vi "Get ESC Ready.vi"(3 "Error in":errorcluster) -> (0 "Error out":errorcluster, 2 "Current PWM%":dbl)   [LabVIEW 2021]
uses:
  Anemometry/Anemometry Sub Vis/Gen Trav/Multi_Run_Status.ctl
  Anemometry/Anemometry Sub Vis/Globals/Meas_global.vi
  Anemometry/Anemometry Sub Vis/Globals/Trav_pos_global.vi
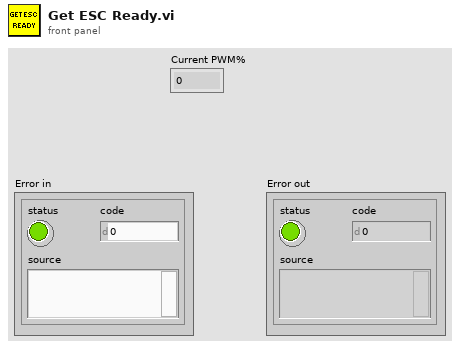
[diagram p1: front panel]
types:
  T1 = typedef "Multi_Run_Status.ctl" = enum16{"Continue", "Continue with Error", "Jump to Next Point", "Jump to Next Row", "Jump To Fall Back", "Terminate Run"}
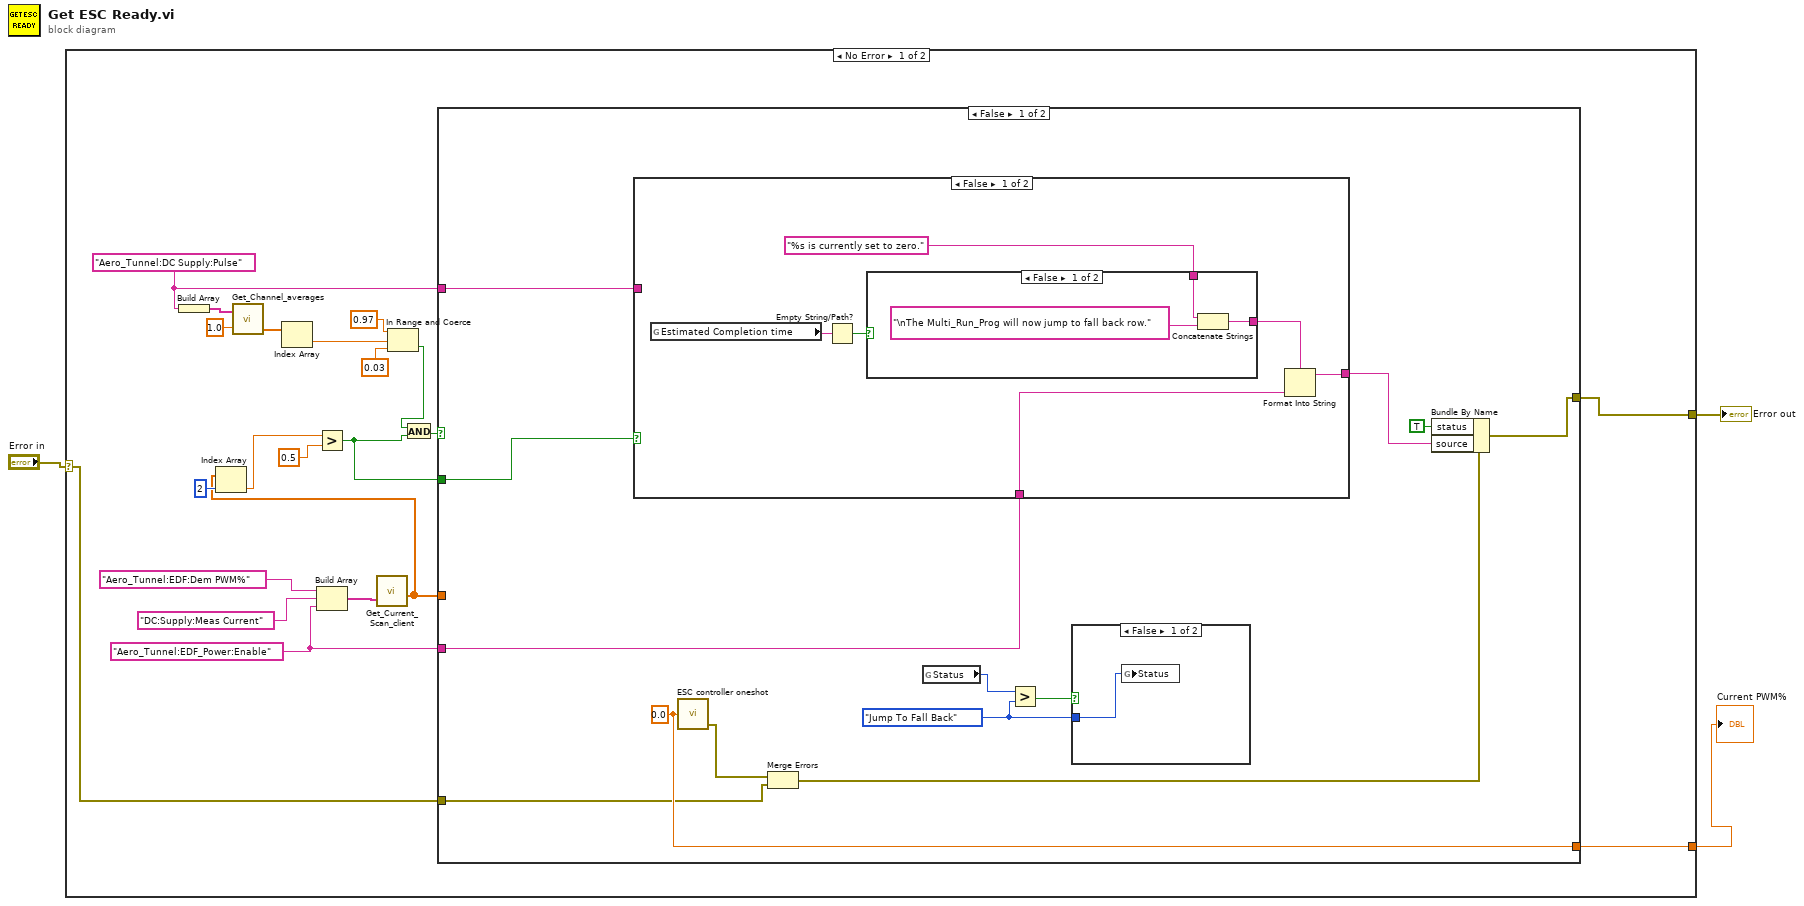
[diagram p0: block diagram]
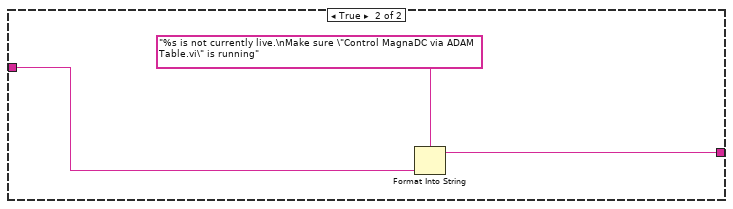
[diagram p3: hidden frame]
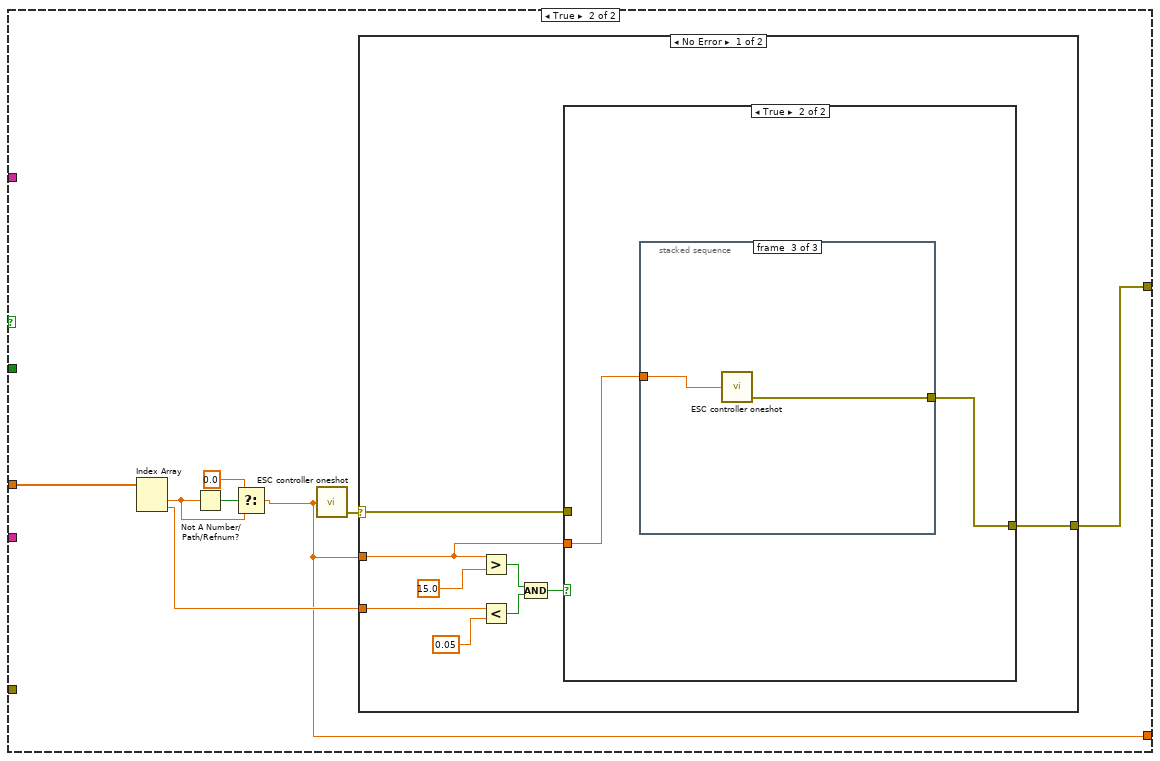
[diagram p5: hidden frame]
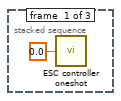
[diagram p7: hidden frame]
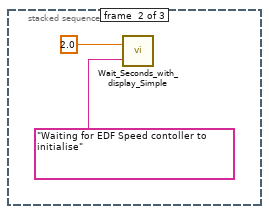
[diagram p8: hidden frame]
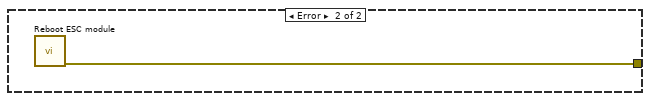
[diagram p9: hidden frame]
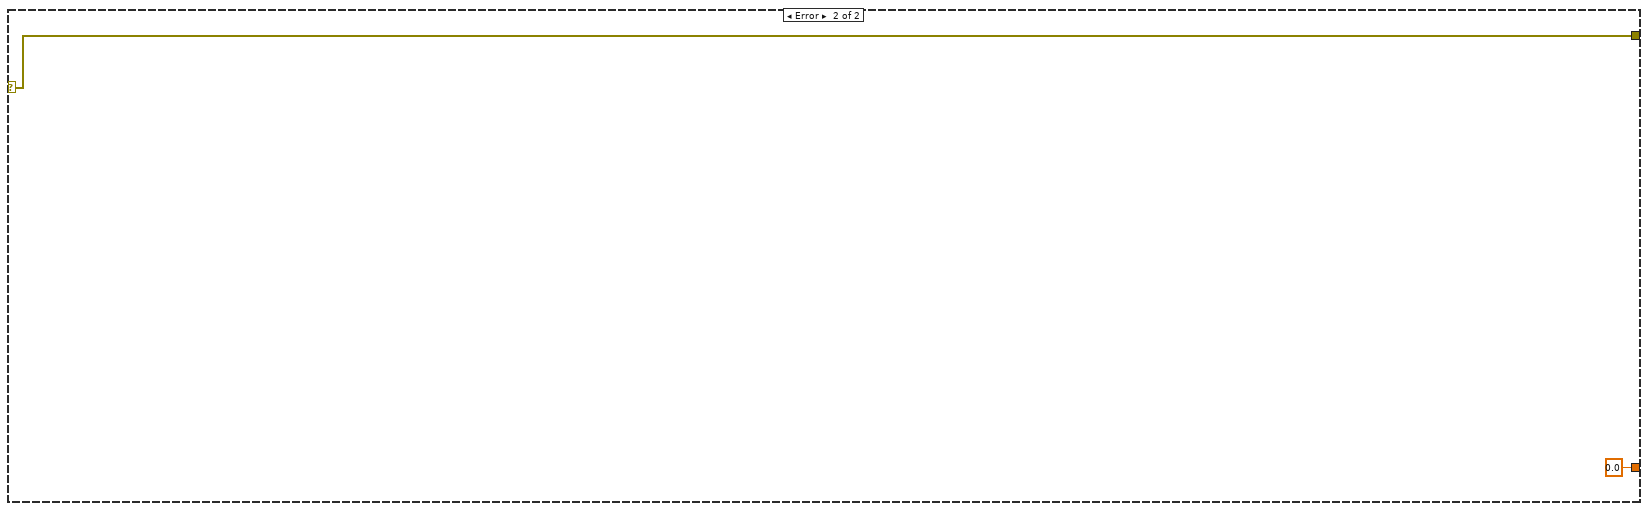
[diagram p10: hidden frame]
diagram:
  n1 = case shown="No Error" "Error in" {
    selector: "Error in" -> [w17 w79]
    tunnel: [w13 w79] -> w2
    tunnel: [w12 0.0 ("t")] -> w1
    frame No Error {
      w4 = "Aero_Tunnel:EDF_Power:Enable"
      w18 = "Aero_Tunnel:DC Supply:Pulse"
      n2 = Build Array(w18) -> (w24:string[])
      n3 = call "Get_Channel_averages.vi"("Desired Ch Names"=w24, "Averaging time (mins)"=1.0) -> ("number"=w23:dbl[])  [unwired: 1 in, 2 out]
      n4 = Index Array(array=w23) -> (element=w22:dbl)  [unwired: 1 in]
      n5 = Build Array("Aero_Tunnel:EDF:Dem PWM%", "DC:Supply:Meas Current", w4) -> (w14:string[])
      n6 = call "Get_Current_Scan_client.vi"("multipleChannels"=w14) -> ("Numerical Values"=w10:dbl[])  [unwired: 1 in, 3 out]
      n7 = Index Array(array=w10, index=2) -> (element=w8:dbl)
      n8 = Greater?(x=w8, y=0.5) -> (0:w5:bool)
      n9 = In Range and Coerce(upper limit=0.97, x=w22, lower limit=0.03) -> (In Range?=w9:bool)  [unwired: 1 out]
      n10 = And(x=w9, y=w5) -> (x .and. y?=w6:bool)
      n11 = case shown="False" w6 {
        tunnel: w18 -> [w34 _]
        tunnel: [w35 w55] -> w13
        tunnel: w17 -> [w26 _]
        tunnel: w10 -> [_ w54]
        tunnel: [w33 w52] -> w12
        tunnel: w5 -> [w29 _]
        tunnel: w4 -> [w28 _]
        frame False {
          w32 = Multi_Run_Status."Jump To Fall Back" ("Status")
          w33 = sgl 0.0 ("Output %")
          n12 = case shown="False" w29 {
            tunnel: [w42 w49] -> w36
            tunnel: w34 -> [_ w48]
            tunnel: w28 -> [w43 _]
            frame False {
              n13 = global read "Trav_pos_global.vi" "Estimated Completion time"() -> (w41:string)
              n14 = Empty String/Path?(string/path=w41) -> (empty?=w40:bool)
              n15 = case shown="False" w40 {
                tunnel: "%s is currently set to zero." ("format string") -> [w46 w47]
                tunnel: [w44 w47] -> w38
                frame False {
                  n16 = Concatenate Strings(w46, "\nThe Multi_Run_Prog will now jump to fall back row." ("string")) -> (w44:string)
                }
                frame True {
                }
              }
              n17 = Format Into String(format string=w38, w43) -> (resulting string=w42:string)  [unwired: 2 in, 1 out]
            }
            frame True {
              n18 = Format Into String(format string="%s is not currently live.\nMake sure \"Control MagnaDC via ADAM Table.vi\" is running", w48) -> (resulting string=w49:string)  [unwired: 2 in, 1 out]
            }
          }
          n19 = call "ESC controller oneshot.vi"("Output %"=w33) -> ("Error out"=w27:errorcluster)  [unwired: 4 in]
          n20 = Merge Errors(w27, w26) -> (w25:errorcluster)
          n21 = global read "Meas_global.vi" "Status"() -> (w30:T1)
          n22 = Greater?(x=w30, y=w32) -> (0:w31:bool)
          n23 = case shown="False" w31 {
            tunnel: w32 -> [w51 _]
            frame False {
              n24 = global write "Meas_global.vi" "Status"(w51) -> ()
            }
            frame True {
            }
          }
          n25 = Bundle By Name(cluster=w25, "status"=TRUE, "source"=w36) -> (w35:errorcluster)
        }
        frame True {
          n26 = Index Array(array=w54) -> (element #1=w58:dbl, element #2=w53:dbl)  [unwired: 2 in]
          n27 = Not A Number/Path/Refnum?(number/path/refnum=w58) -> (NaN/Path/Refnum?=w59:bool)
          n28 = Select(t=0.0, s=w59, f=w58) -> (s? t:f=w52:dbl)
          n29 = call "ESC controller oneshot.vi"("Output %"=w52) -> ("Error out"=w56:errorcluster)  [unwired: 4 in]
          n30 = case shown="No Error" w56 {
            selector: w56 -> [w62 _]
            tunnel: [w63 w77] -> w55
            tunnel: w52 -> [w60 _]
            tunnel: w53 -> [w66 _]
            frame No Error {
              n31 = Greater?(x=w60, y=15.0) -> (0:w65:bool)
              n32 = Less?(x=w66, y=0.05) -> (x < y?=w64:bool)
              n33 = Compound Arithmetic op=AND(w65, w64) -> (w61:bool)
              n34 = case shown="True" w61 {
                tunnel: [w69 w70] -> w63
                tunnel: w62 -> [w69 _]
                tunnel: w60 -> [_ w71]
                frame False {
                }
                frame True {
                  n35 = stacked-sequence {
                    tunnel: w71 -> [_ _ w76]
                    tunnel: [_ _ w75] -> w70
                    frame #0 {
                      n36 = call "ESC controller oneshot.vi"("Output %"=sgl 0.0) -> ()  [unwired: 4 in, 1 out]
                    }
                    frame #1 {
                      n37 = call "Wait_Seconds_with_display_Simple.vi"("Message"="Waiting for EDF Speed contoller to initialise", "Seconds to wait"=2.0) -> ()  [unwired: 1 in, 1 out]
                    }
                    frame #2 {
                      n38 = call "ESC controller oneshot.vi"("Output %"=w76) -> ("Error out"=w75:errorcluster)  [unwired: 4 in]
                    }
                  }
                }
              }
            }
            frame Error {
              n39 = call "Reboot ESC module.vi"() -> ("Error out"=w77:errorcluster)  [unwired: 11 in]
            }
          }
        }
      }
    }
    frame Error {
    }
  }
  "Error out" <- w2
  "Current PWM%" <- w1
